vi "gl_Queues.vi"() -> ()   [LabVIEW 2013]
uses:
  User Interface/Queue/Message Queue/Typedefs/All Message Queues.ctl
  User Interface/Queue/Message Queue/Typedefs/Message Cluster.ctl
  Typedefs/Logging queue element.ctl
  Typedefs/Imaging Protocols enum.ctl
  Typedefs/Frame Size.ctl
  Typedefs/Acquired points count.ctl
panel:
  in  "UI queue name":string="UI Queue"
  out "Queues Cluster":T1
  # "e"
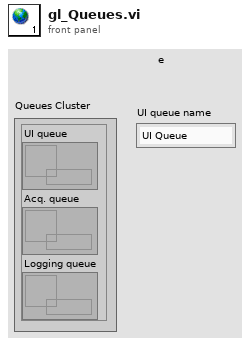
[diagram p1: front panel]
types:
  T1 = typedef "All Message Queues.ctl" = cluster{"UI queue":refnum<queue>, "Acq. queue":refnum<queue>, "Logging queue":refnum<queue>}
diagram:
